vi "S2C_VAR_Initialize.vi"(8 "Error In":errorcluster, 11 "CtrlRef":refnum<vi>) -> (0 "Error Out":errorcluster)   [LabVIEW 2015]
uses:
  S2C_VAR_Globals.vi
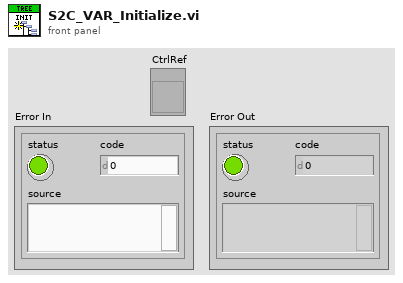
[diagram p1: front panel]
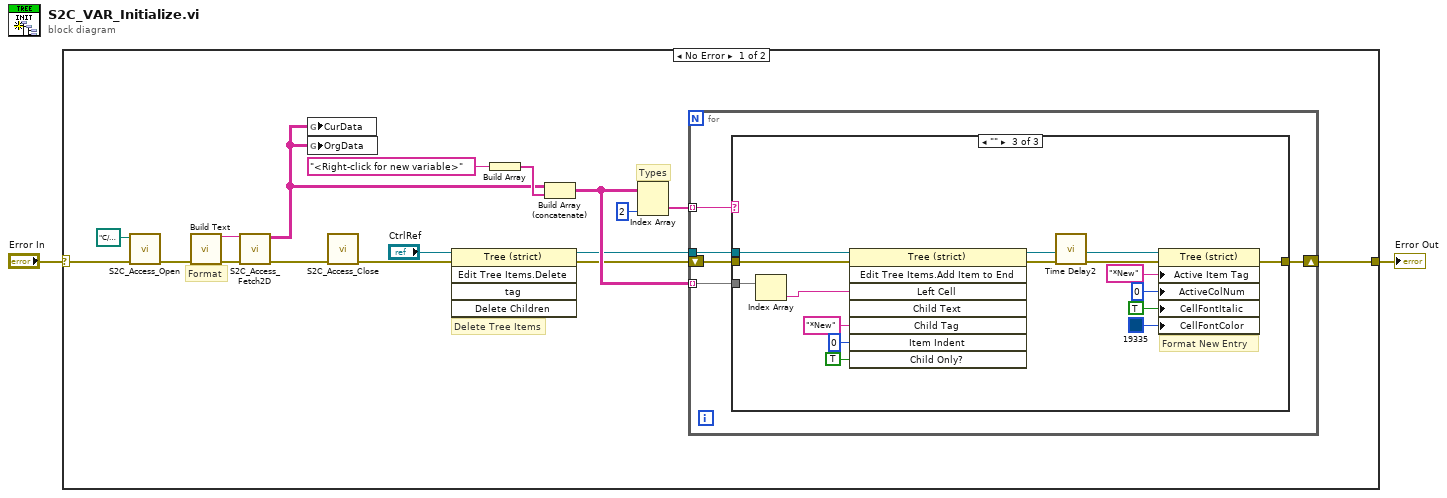
[diagram p0: block diagram]
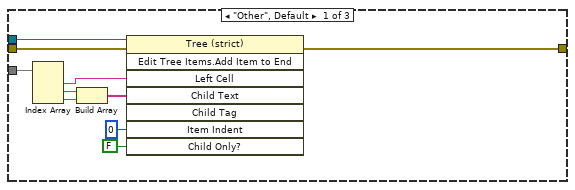
[diagram p2: hidden frame]
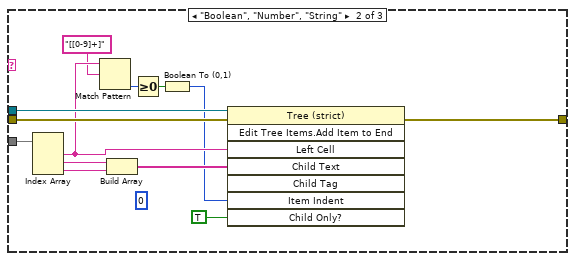
[diagram p3: hidden frame]
diagram:
  n1 = case shown="No Error" "Error In" {
    selector: "Error In" -> [w19 w63]
    tunnel: [w9 w63] -> w1
    frame No Error {
      # "Format"
      # "Types"
      # "Delete Tree Items"
      n2 = call "S2C_Access_Open.vi"("Error In"=w19, "DSN_Path"=path "C:/Personal/Labview/S2C/AccessDB.dsn") -> ("Error Out"=w7:errorcluster)  [unwired: 8 in, 1 out]
      n3 = call "Build Text"("error in (no error)"=w7) -> ("Result"=w5:string, "error out"=w6:errorcluster)  [unwired: 13 in]
      n4 = call "S2C_Access_Fetch2D.vi"("Error In"=w6, "Query"=w5) -> ("Error Out"=w4:errorcluster, "Data"=w3:string[][])  [unwired: 8 in]
      n5 = global write "S2C_VAR_Globals.vi" "CurData"(w3) -> ()
      n6 = global write "S2C_VAR_Globals.vi" "OrgData"(w3) -> ()
      n7 = call "S2C_Access_Close.vi"("Error In"=w4) -> ("Error Out"=w12:errorcluster)  [unwired: 10 in]
      n8 = invoke on="Invoke Node" class="Tree (strict)" method="Edit Tree Items.Delete"(reference="CtrlRef", error in=w12) -> (reference out=w10:refnum<vi>, error out=w11:errorcluster)  [unwired: 3 in, 3 out]
      n9 = Build Array("<Right-click for new variable>") -> (w15:string[])
      n10 = Build Array (concatenate)(w3, w15) -> (w14:string[][])
      n11 = Index Array(array=w14, index (col)=2 ("disabled index (col)")) -> (element=w17:string[])  [unwired: 1 in]
      n12 = for {
        tunnel: w14 -> [w22] mode=indexing
        tunnel: w17 -> [w23] mode=indexing
        shift-right: [w21] -> w9
        shift-left: w11 -> [w24]
        tunnel: w10 -> [w20]
        n13 = case shown="\"\"" w23 {
          tunnel: w24 -> [w34 w47 w62]
          tunnel: w22 -> [w33 w46 w61]
          tunnel: [w25 w40 w49] -> w21
          tunnel: w20 -> [w26 w41 w48]
          frame "Other", Default {
            n14 = Index Array(array=w33) -> (element #1=w30:string, element #2=w32:string, element #3=w31:string)  [unwired: 3 in]
            n15 = Build Array(w32, w31) -> (w29:string[])
            n16 = invoke on="Invoke Node" class="Tree (strict)" method="Edit Tree Items.Add Item to End"(reference=w26, error in=w34, "Left Cell"=w30, "Child Text"=w29, "Item Indent"=0 ("New Item Indentation"), "Child Only?"=FALSE) -> (error out=w25:errorcluster)  [unwired: 2 in, 7 out]
          }
          frame "Boolean", "Number", "String" {
            (unwired) 0 ("New Item Indentation")
            n17 = Index Array(array=w46) -> (element #1=w39:string, element #2=w45:string, element #3=w44:string)  [unwired: 3 in]
            n18 = Match Pattern(string=w39, regular expression="[[0-9]+]" ("string")) -> (offset past match=w37:i32)  [unwired: 1 in, 3 out]
            n19 = Build Array(w45, w44) -> (w43:string[])
            n20 = Greater Or Equal To 0?(x=w37) -> (x >= 0?=w36:bool)
            n21 = Boolean To (0,1)(Boolean=w36) -> (0, 1=w35:i16)
            n22 = invoke on="Invoke Node" class="Tree (strict)" method="Edit Tree Items.Add Item to End"(reference=w41, error in=w47, "Left Cell"=w39, "Child Text"=w43, "Item Indent"=w35, "Child Only?"=TRUE) -> (error out=w40:errorcluster)  [unwired: 2 in, 7 out]
          }
          frame "" {
            # "Format New Entry"
            n23 = Index Array(array=w61) -> (element=w60:string)  [unwired: 1 in]
            n24 = invoke on="Invoke Node" class="Tree (strict)" method="Edit Tree Items.Add Item to End"(reference=w48, error in=w62, "Left Cell"=w60, "Child Tag"="*New", "Item Indent"=0 ("New Item Indentation"), "Child Only?"=TRUE) -> (reference out=w51:refnum<vi>, error out=w50:errorcluster)  [unwired: 2 in, 6 out]
            n25 = call "Time Delay2"("error in (no error)"=w50) -> ("error out"=w52:errorcluster)  [unwired: 10 in]
            n26 = property on="Property Node" class="Tree (strict)"(reference=w51, error in=w52, "Active Item Tag"="*New", "ActiveColNum"=0 ("Active Cell:Active Column Number"), "CellFontItalic"=TRUE ("Active Cell:Cell Font:Italic"), "CellFontColor"=u32 19335) -> (error out=w49:errorcluster)  [unwired: 1 out]
          }
        }
      }
    }
    frame Error {
    }
  }
  "Error Out" <- w1
